vi "Unregister Process.vi"(0 "Message Handler In":refnum<class "Message Handler.lvclass">, 7 "Process":refnum<class "ICanCommunicate.lvclass">, 11 "Error In":errorcluster) -> (4 "Message Handler Out":refnum<class "Message Handler.lvclass">, 15 "Error Out":errorcluster)   [LabVIEW 2023, in "Message Handler.lvclass"]
uses:
  Message Handler.lvclass
  Interfaces/ICanCommunicate/ICanCommunicate.lvclass
  Interfaces/ICanCommunicate/Message.ctl
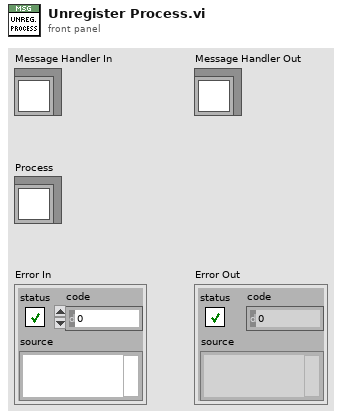
[diagram p1: front panel]
types:
  T1 = typedef "ICanCommunicate.lvclass/Message.ctl" = cluster{"Sender Name":string, "Recipent Name":string, "Command":string, "Data":variant, "Signature":string}
  T2 = typedef "ICanCommunicate.lvclass/ToProcessQueue.ctl" = refnum<queue>
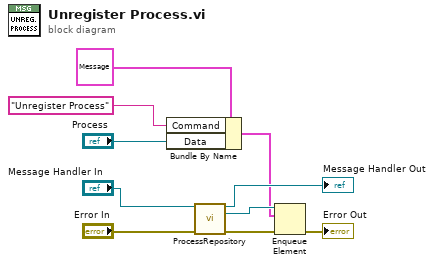
[diagram p0: block diagram]
diagram:
  n1 = Bundle By Name(cluster=T1 {"Sender Name"="", "Recipent Name"="", "Command"="", "Data"=variant, "Signature"=""} ("Message"), "Command"="Unregister Process", "Data"="Process") -> (w5:T1)
  n2 = call-dynamic "ProcessRepository.vi"("Process In"="Message Handler In", "Error In"="Error In") -> ("Process Out"=→"Message Handler Out":refnum<class "Message Handler.lvclass">, "ToProcessQueue"=w8:T2, "Error Out"=w4:errorcluster)  [unwired: 7 in, 4 out]
  n3 = Enqueue Element(queue=w8, element=w5, error in (no error)=w4) -> (error out=→"Error Out":errorcluster)  [unwired: 1 in, 2 out]
